vi "题目6.3.vi"() -> ()   [LabVIEW 2017]
uses:
  <vilib>/measure/NI_MABase.lvlib
panel:
  in  "基路径":path
  out "Y":dbl[](array[numeric])
  in  "phase":dbl caption="相位" format="%.2p"
  in  "amplitude":dbl=1.0 caption="幅值" format="%0.2p"
  in  "frequency":dbl=10.0 caption="频率" format="%0.2p"
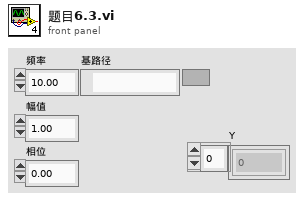
[diagram p1: front panel]
types:
  T1 = enum16{"open", "replace", "create", "open or create", "replace or create", "replace or create with confirmation"}
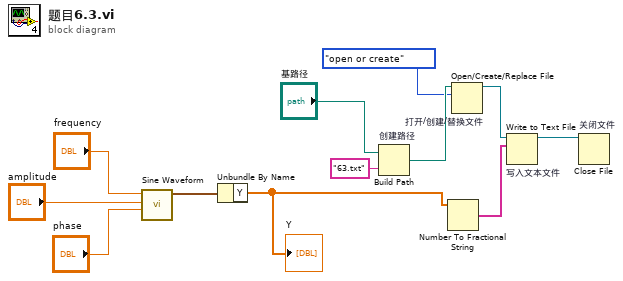
[diagram p0: block diagram]
diagram:
  n1 = call <vilib>:"Sine Waveform.vi"("phase"="phase", "amplitude"="amplitude", "frequency"="frequency") -> ("signal out"=w9:waveform(dbl))  [unwired: 7 in, 1 out]
  n2 = Unbundle By Name(w9) -> ("Y"=w6:dbl[])
  "Y" <- w6
  n3 = Build Path "创建路径"(base path="基路径", name or relative path="63.txt" ("名称或相对路径")) -> (appended path=w5:path)
  n4 = Number To Fractional String(number=w6) -> (F-format string=w2:string[])  [unwired: 3 in]
  n5 = Open/Create/Replace File "打开/创建/替换文件"(file path (use dialog)=w5, operation (0:open)=T1."open or create" ("操作(0:open)")) -> (refnum out=w1:refnum<file>)  [unwired: 4 in, 2 out]
  n6 = Write to Text File "写入文本文件"(file (use dialog)=w1, text=w2) -> (refnum out=w3:refnum<file>)  [unwired: 2 in, 2 out]
  n7 = Close File "关闭文件"(refnum=w3) -> ()  [unwired: 1 in, 2 out]
